vi "CRYGet Channel Array ASIO.vi"(11 "Channel Array":T1[](array[typedef]) {"Coupling" items=["Default"=-1, "RSE"=10083, "NRSE"=10078, "Differential"=10106, "Pseudodifferential"=12529]; "term config" items=["Default"=-1, "RSE"=10083, "NRSE"=10078, "Differential"=10106, "Pseudodifferential"=12529]; "Anti-aliasing Factor (%fs)" format="%.2f"}) -> (0 "I Channel Info Out":T1[](array[typedef]) {"Coupling" items=["Default"=-1, "RSE"=10083, "NRSE"=10078, "Differential"=10106, "Pseudodifferential"=12529]; "term config" items=["Default"=-1, "RSE"=10083, "NRSE"=10078, "Differential"=10106, "Pseudodifferential"=12529]; "Anti-aliasing Factor (%fs)" format="%.2f"}, 1 "I Channel Name Out":string[](array[string]), 2 "O Channel Info Out":T1[](array[typedef]) {"Coupling" items=["Default"=-1, "RSE"=10083, "NRSE"=10078, "Differential"=10106, "Pseudodifferential"=12529]; "term config" items=["Default"=-1, "RSE"=10083, "NRSE"=10078, "Differential"=10106, "Pseudodifferential"=12529]; "Anti-aliasing Factor (%fs)" format="%.2f"}, 3 "O Channel Name Out":string[](array[string]))   [LabVIEW 2013]
uses:
  Typedef Control/CRYHardware Channel Info.ctl
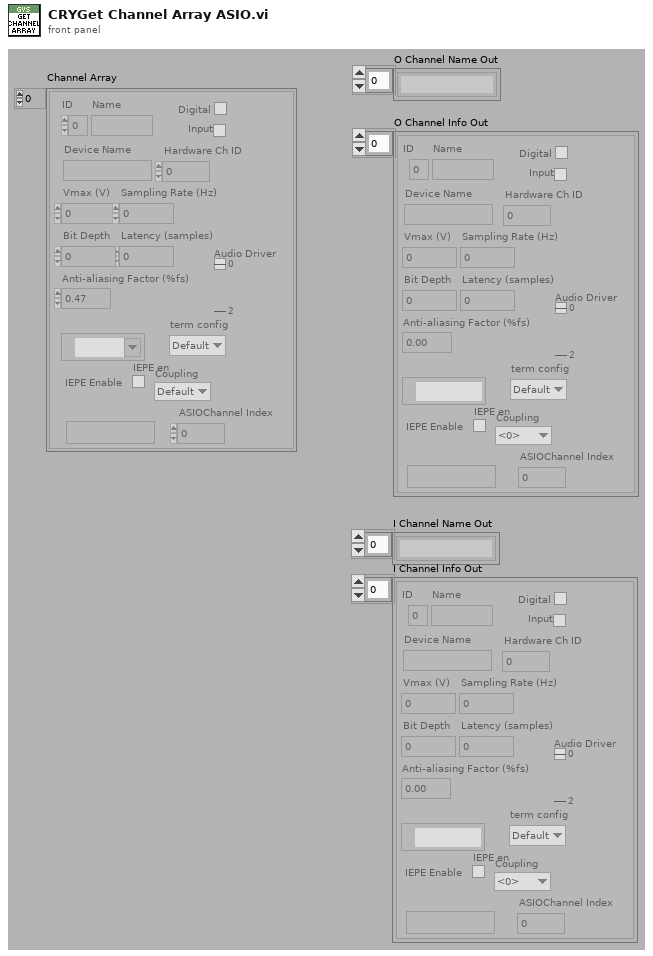
[diagram p1: front panel]
types:
  T1 = typedef "CRYHardware Channel Info.ctl" = cluster{"ID":i32, "Name":string, "Digital":bool, "Input":bool, "Device Name":string, "Hardware Ch ID":u8, "Vmax (V)":dbl, "Latency (samples)":dbl, "Sampling Rate (Hz)":u32, "Bit Depth":u32, "Anti-aliasing Factor (%fs)":sgl, "DAQmx Channel":tag, "term config":i32, "Coupling":i32, "IEPE en":bool, "ASIOChannel Name":string, "Audio Driver":u16, "ASIOChannel Index":u8}
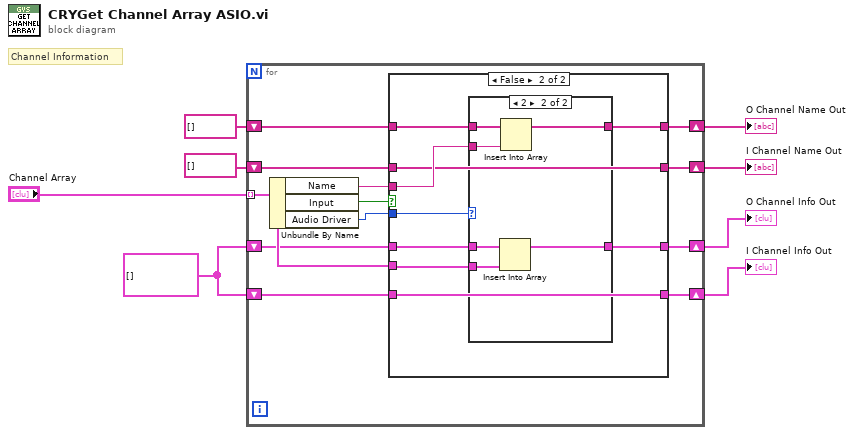
[diagram p0: block diagram]
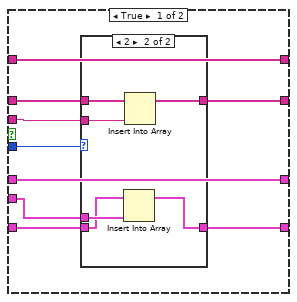
[diagram p2: hidden frame]
diagram:
  w6 = T1[] []
  # "Channel Information"
  n1 = for {
    tunnel: "Channel Array" -> [w14] mode=indexing
    shift-right: [w19] -> w5
    shift-left: string[] [] -> [w18]
    shift-right: [w15] -> w4
    shift-left: string[] [] -> [w16]
    shift-right: [w13] -> w3
    shift-left: w6 -> [w12]
    shift-right: [w11] -> w2
    shift-left: w6 -> [w10]
    n2 = Unbundle By Name(w14) -> ("Name"=w20:string, "Input"=w17:bool, "Audio Driver"=w9:u16)
    n3 = case shown="False" w17 {
      tunnel: w20 -> [w29 w46]
      tunnel: [w26 w45] -> w19
      tunnel: w18 -> [w26 w44]
      tunnel: w16 -> [w28 w43]
      tunnel: [w27 w43] -> w15
      tunnel: w14 -> [w24 w42]
      tunnel: [w25 w41] -> w13
      tunnel: w12 -> [w25 w40]
      tunnel: [w23 w39] -> w11
      tunnel: w10 -> [w22 w39]
      tunnel: w9 -> [w21 w38]
      frame True {
        n4 = case shown="2" w21 {
          tunnel: w29 -> [_ w37]
          tunnel: w28 -> [w31 w36]
          tunnel: [w31 w35] -> w27
          tunnel: w24 -> [_ w34]
          tunnel: [w30 w33] -> w23
          tunnel: w22 -> [w30 w32]
          frame Default {
          }
          frame 2 {
            n5 = Insert Into Array(array=w32, new element=w34) -> (w33:T1[])  [unwired: 1 in]
            n6 = Insert Into Array(array=w36, new element=w37) -> (w35:string[])  [unwired: 1 in]
          }
        }
      }
      frame False {
        n7 = case shown="2" w38 {
          tunnel: w46 -> [_ w54]
          tunnel: [w48 w53] -> w45
          tunnel: w44 -> [w48 w52]
          tunnel: w42 -> [_ w51]
          tunnel: [w47 w50] -> w41
          tunnel: w40 -> [w47 w49]
          frame Default {
          }
          frame 2 {
            n8 = Insert Into Array(array=w49, new element=w51) -> (w50:T1[])  [unwired: 1 in]
            n9 = Insert Into Array(array=w52, new element=w54) -> (w53:string[])  [unwired: 1 in]
          }
        }
      }
    }
  }
  "O Channel Name Out" <- w5
  "I Channel Name Out" <- w4
  "O Channel Info Out" <- w3
  "I Channel Info Out" <- w2
